vi "Update FIFO State - 32-bit Address.vi"(0 "issue write":bool, 1 "reset":bool, 5 "fifo depth":T2=8 items=["4"=2, "8"=3, "16"=4, "32"=5, "64"=6, "128"=7, "256"=8, "512"=9, "1024"=10, "2048"=11, "4096"=12, "8192"=13, "16384"=14, "32768"=15, "65536"=16, "131072"=17, "262144"=18, "524288"=19, "1048576"=20, "2097152"=21, "4194304"=22, "8388608"=23, "16777216"=24, "33554432"=25, "67108864"=26, "134217728"=27, "268435456"=28, "536870912"=29, "1073741824"=30, "2147483648"=31, "4294967296"=32], 12 "ready for read request":bool) -> (4 "state":T1, 6 "issue read request":bool, 14 "ready for write":bool)   [LabVIEW 2012, in "FIFO.lvlib"]
uses:
  <userlib>/FPGA Library/Code Development/DRAM/RF-RIO/FIFO/FIFO/FPGA/FIFO.lvlib
  <userlib>/FPGA Library/Code Development/DRAM/RF-RIO/FIFO/FIFO/FPGA/Private/FIFO Depth - 32-bit Address.ctl
  <userlib>/FPGA Library/Code Development/DRAM/RF-RIO/FIFO/FIFO/FPGA/Private/FIFO State - 32-bit Address.ctl
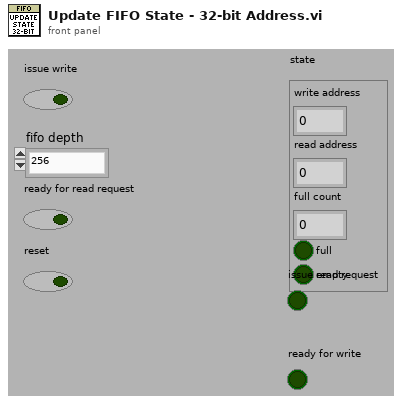
[diagram p1: front panel]
types:
  T1 = typedef "FIFO.lvlib/FIFO State - 32-bit Address.ctl" = cluster{"write address":u32, "read address":u32, "full count":u32, "full":bool, "empty":bool}
  T2 = typedef "FIFO.lvlib/FIFO Depth - 32-bit Address.ctl" = u8
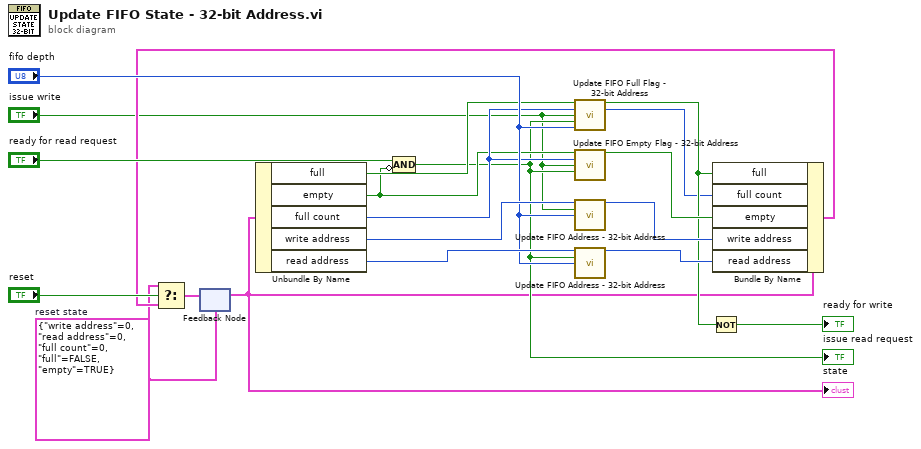
[diagram p0: block diagram]
diagram:
  w1 = T1 {"write address"=0, "read address"=0, "full count"=0, "full"=FALSE, "empty"=TRUE}  # reset state
  n1 = feedback #1(w1) -> (w3:T1)
  "state" <- w3
  n2 = Unbundle By Name(w3) -> ("full"=w13:bool, "empty"=w12:bool, "full count"=w14:u32, "write address"=w20:u32, "read address"=w19:u32)
  n3 = Compound Arithmetic op=AND("ready for read request", invert w12) -> (w8:bool)
  "issue read request" <- w8
  n4 = call <userlib>:"Update FIFO Full Flag - 32-bit Address.vi"("full in"=w13, "full count in"=w14, "write"="issue write", "read"=w8, "fifo depth"="fifo depth") -> ("full out"=w10:bool, "full count out"=w7:u32)  [unwired: 9 in]
  n5 = call <userlib>:"Update FIFO Empty Flag - 32-bit Address.vi"("empty in"=w12, "full count"=w14, "write"="issue write", "read"=w8) -> ("empty out"=w15:bool)  [unwired: 11 in]
  n6 = call <userlib>:"Update FIFO Address - 32-bit Address.vi"("address in"=w20, "increment"="issue write", "fifo depth"="fifo depth") -> ("address out"=w18:u32)  [unwired: 12 in]
  n7 = call <userlib>:"Update FIFO Address - 32-bit Address.vi"("address in"=w19, "increment"=w8, "fifo depth"="fifo depth") -> ("address out"=w17:u32)  [unwired: 12 in]
  n8 = Not(x=w10) -> (.not. x?=→"ready for write":bool)
  n9 = Bundle By Name(cluster=w3, "full"=w10, "full count"=w7, "empty"=w15, "write address"=w18, "read address"=w17) -> (w4:T1)
  n10 = Select(t=w1, s="reset", f=w4) -> (s? t:f=w5:T1)
  n11 = feedback-in #1(w5) -> ()
